vi "shift register in while loop.vi"() -> ()   [LabVIEW 2016]
panel:
  in  "stop":bool
  out "Three Iterations Ago":i32
  out "Two Iterations Ago":i32
  out "Previous Count":i32
  out "Current Count":i32
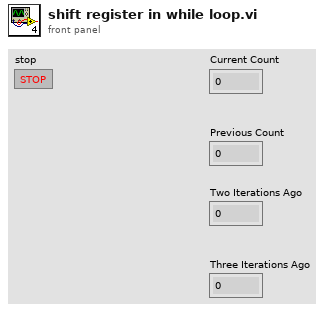
[diagram p1: front panel]
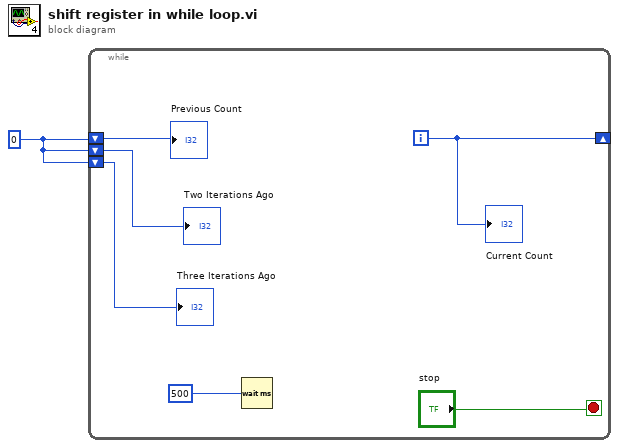
[diagram p0: block diagram]
diagram:
  w1 = 0
  n1 = while {
    shift-right: [w7] -> _
    shift-left: w1 -> [w6]
    shift-left: w1 -> [w5]
    shift-left: w1 -> [w4]
    i -> [w7]
    stop <- "stop" stop-if-true
    n2 = Wait (ms)(milliseconds to wait=u32 500 ("millisecond timer value")) -> ()  [unwired: 1 out]
    "Current Count" <- w7
    "Previous Count" <- w6
    "Two Iterations Ago" <- w5
    "Three Iterations Ago" <- w4
  }
